vi "fil ter.vi"(8 "path":string, 9 "multiplication/ substitution":i16(ring) items=["subst", "mult"], 10 "intensity / phase":i16(ring) items=["int", "pha"], 11 "field":T1) -> (0 "Path Filter":string, 3 "field out":T1)   [LabVIEW 2012, in "LightPipes.lvlib"]
doc: "__declspec(dllexport) void fil_ter(FIELD* field, const char* data, const char* c1, const char* c2);\n\n__declspec(dllexport) void fil_ter(FIELD* field, const char* path, const char* c1, const char* c2);"
uses:
  LightPipes.lvlib
  <userlib>/LightPipes/LightPipes.dll
panel:
  out "error out":errorcluster
  # "@param c1:    the c1 option (int, pha)\n@param c2:    the c2 option (mult, subst)"
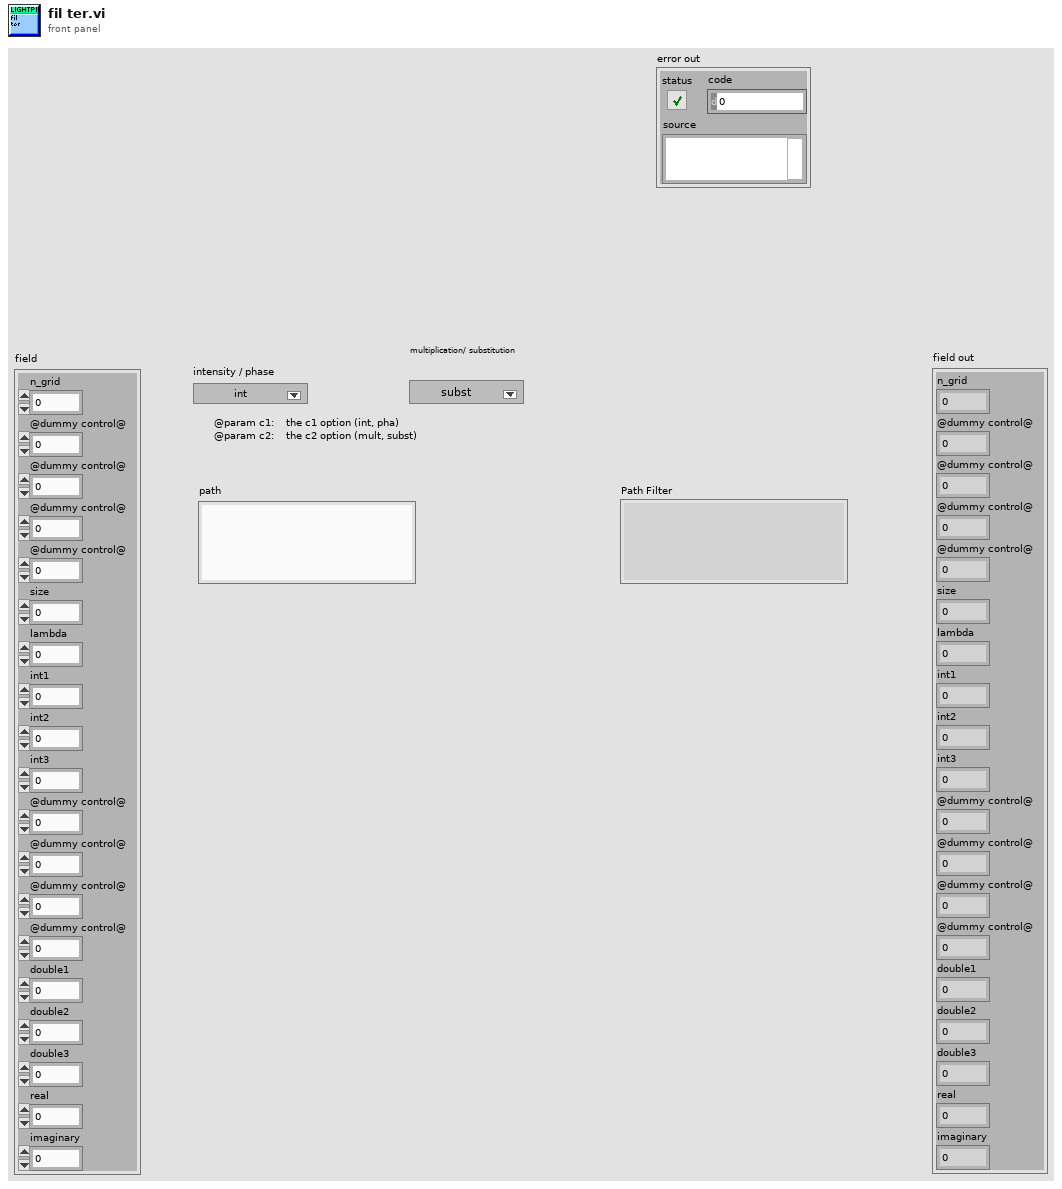
[diagram p1: front panel]
types:
  T1 = cluster{"n_grid":i32, "@dummy control@":i8, "@dummy control@":i8, "@dummy control@":i8, "@dummy control@":i8, "size":dbl, "lambda":dbl, "int1":i32, "int2":i32, "int3":i32, "@dummy control@":i8, "@dummy control@":i8, "@dummy control@":i8, "@dummy control@":i8, "double1":dbl, "double2":dbl, "double3":dbl, "real":u32, "imaginary":u32}
  T2 = enum16{"open", "replace", "create", "open or create", "replace or create", "replace or create with confirmation"}
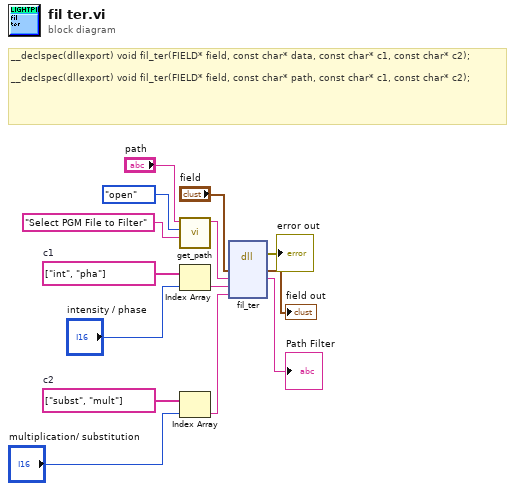
[diagram p0: block diagram]
diagram:
  w9 = string[] ["int", "pha"]  # c1
  w12 = string[] ["subst", "mult"]  # c2
  # "__declspec(dllexport) void fil_ter(FIELD* field, const char* data, const char* c1, const char* c2);\n\n__declspec(dllexport) void fil_ter(FIELD* field, const char* path, const char* c1, const char* c2);"
  n1 = call "get_path.vi"("Message Prompt"="Select PGM File to Filter", "operation (default: open/create)"=T2."open" ("operation (0:open)"), "Path in"="path") -> ("Path out"=w4:string)  [unwired: 8 in]
  n2 = Index Array(array=w9, index="intensity / phase") -> (element=w7:string)
  n3 = Index Array(array=w12, index="multiplication/ substitution") -> (element=w10:string)
  n4 = dll-call lib="C:/Program Files (x86)/National Instruments/LabVIEW 2012/user.lib/LightPipes/LightPipes.*" fn="fil_ter"("field"="field", "path"=w4, "c1"=w7, "c2"=w10) -> (error out=→"error out":errorcluster, "field"=→"field out":T1, "path"=→"Path Filter":string)  [unwired: 6 in, 1 out]
